vi "ExecuteSpeed.vi"(8 "Error In":errorcluster, 11 "RobotDriveDevRef":T1={"DevStatus"={"status"=FALSE, "code"=0, "source"=""}, "Motors[]"=[], "Square Inputs"=FALSE, "Max Output"=1.0}) -> (0 "Error Out":errorcluster)   [LabVIEW 2020]
uses:
  <vilib>/Rock Robotics/WPI/RobotDrive/WPI_RobotDriveDevRef.ctl
  <vilib>/Rock Robotics/WPI/MotorControl/WPI_MotorControlDeviceRef.ctl
  <vilib>/Rock Robotics/WPI/MotorControl/WPI_MotorControlType.ctl
  <vilib>/Rock Robotics/SystemInterfaces/DIO/FPGA_DIOPWMChannel.ctl
  <vilib>/Rock Robotics/WPI/PWM/WPI_PWMDeadband.ctl
  <vilib>/Rock Robotics/SystemInterfaces/DIO/FPGA_DIOChannel.ctl
  <vilib>/Rock Robotics/WPI/ThirdParty/JAS_Junk/TrajLib/PIDController_AtSetpoint.vi
  <vilib>/Rock Robotics/WPI/ThirdParty/JAS_Junk/TrajLib/PIDController_SetPIDF.vi
  <vilib>/Rock Robotics/WPI/ThirdParty/JAS_Junk/TrajLib/PIDController_SetDerivativeFilter.vi
  <vilib>/Rock Robotics/WPI/ThirdParty/JAS_Junk/TrajLib/PIDController_SetIntegratorRange.vi
  <vilib>/Rock Robotics/WPI/ThirdParty/JAS_Junk/TrajLib/PIDController_SetTolerancePandV.vi
  <vilib>/Rock Robotics/WPI/ThirdParty/JAS_Junk/TrajLib/PIDController_DisableContinousInput.vi
  <vilib>/Rock Robotics/WPI/ThirdParty/JAS_Junk/TrajLib/PIDController_EnableContinousInput.vi
  <vilib>/Rock Robotics/WPI/ThirdParty/JAS_Junk/TrajLib/PIDController_Reset.vi
  <vilib>/Rock Robotics/WPI/ThirdParty/JAS_Junk/TrajLib/PIDController_New.vi
  <vilib>/Rock Robotics/WPI/ThirdParty/JAS_Junk/TrajLib/PIDController_SetOutputLimits.vi
  <vilib>/Rock Robotics/WPI/ThirdParty/JAS_Junk/TrajLib/SlewRateLimiter_New.vi
  <vilib>/Rock Robotics/WPI/ThirdParty/JAS_Junk/TrajLib/SlewRateLimiter_Reset.vi
  <vilib>/Rock Robotics/WPI/ThirdParty/JAS_Junk/TrajLib/SlewRateLimiter_Calculate.vi
  <vilib>/Rock Robotics/WPI/ThirdParty/JAS_Junk/TrajLib/SlewRateLimiter_SetRate.vi
  <vilib>/Rock Robotics/WPI/ThirdParty/JAS_Junk/TrajLib/ControllerUtil_GetModulusError.vi
  <vilib>/Rock Robotics/WPI/ThirdParty/JAS_Junk/TrajLib/PIDController_NewPeriod.vi
  <vilib>/Rock Robotics/SystemInterfaces/NetworkCommunication/NetComm_UsageReport_report.vi
  DriveGlobals.vi
  <vilib>/Rock Robotics/WPI/ThirdParty/JAS_Junk/TrajLib/Util_GetTime.vi
  <vilib>/Rock Robotics/WPI/ThirdParty/JAS_Junk/TrajLib/Util_LibraryGlobals.vi
  <vilib>/Rock Robotics/WPI/ThirdParty/JAS_Junk/TrajLib/PIDController_AdvCalculate_FF_Sp_Pv.vi
  <vilib>/Rock Robotics/Network Tables/NT Write Numeric Array.vi
  <vilib>/Rock Robotics/WPI/ThirdParty/JAS_Junk/TrajLib/Trajectory_Library.lvlib
  <vilib>/Rock Robotics/WPI/DriverStation/WPI_DriverStationRobotMode2.ctl
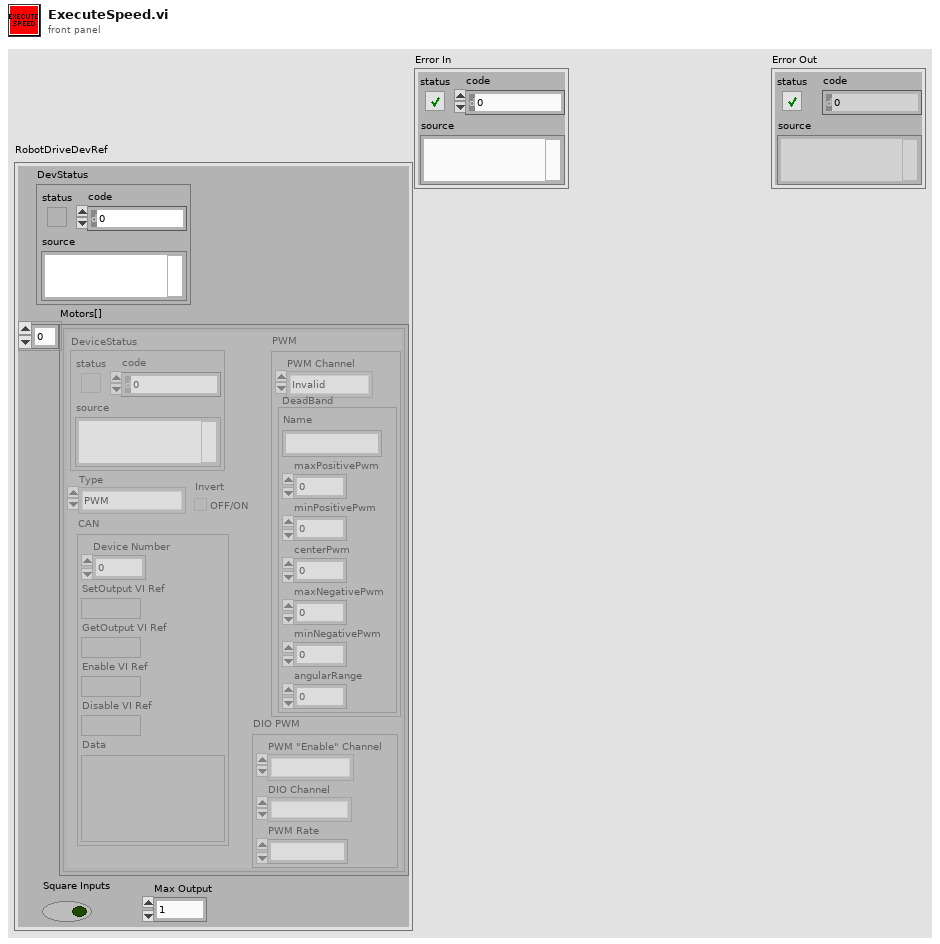
[diagram p1: front panel]
types:
  T1 = typedef "WPI_RobotDriveDevRef.ctl" = cluster{"DevStatus":errorcluster, "Motors[]":T2[], "Square Inputs":bool, "Max Output":dbl}
  T2 = typedef "WPI_MotorControlDeviceRef.ctl" = cluster{"DeviceStatus":errorcluster, "Type":T3, "PWM":cluster{"PWM Channel":T4, "DeadBand":T5}, "CAN":cluster{"Device Number":u8, "SetOutput VI Ref":variant, "GetOutput VI Ref":variant, "Enable VI Ref":variant, "Disable VI Ref":variant, "Data":variant}, "Invert":bool, "DIO PWM":cluster{"PWM \"Enable\" Channel":T4, "DIOChannel":T6, "PWM Rate":dbl}}
  T3 = typedef "WPI_MotorControlType.ctl" = enum16{"PWM", "CAN", "DIO PWM"}
  T4 = typedef "FPGA_DIOPWMChannel.ctl" = enum8{"PWM 0", "PWM 1", "PWM 2", "PWM 3", "PWM 4", "PWM 5", "PWM 6", "PWM 7", "PWM 8", "PWM 9", "PWM MXP 0", "PWM MXP 1", "PWM MXP 2", "PWM MXP 3", "PWM MXP 4", "PWM MXP 5", "PWM MXP 6", "PWM MXP 7", "PWM MXP 8", "PWM MXP 9", "Invalid"}
  T5 = typedef "WPI_PWMDeadband.ctl" = cluster{"Name":string, "maxPositivePwm":i32, "minPositivePwm":i32, "centerPwm":i32, "maxNegativePwm":i32, "minNegativePwm":i32, "angularRange":u16}
  T6 = typedef "FPGA_DIOChannel.ctl" = enum8{"DIO 0", "DIO 1", "DIO 2", "DIO 3", "DIO 4", "DIO 5", "DIO 6", "DIO 7", "DIO 8", "DIO 9", "DIO MXP 0", "DIO MXP 1", "DIO MXP 2", "DIO MXP 3", "DIO MXP 4", "DIO MXP 5", "DIO MXP 6", "DIO MXP 7", "DIO MXP 8", "DIO MXP 9", "DIO MXP 10", "DIO MXP 11", "DIO MXP 12", "DIO MXP 13", "DIO MXP 14", "DIO MXP 15", "SPI Port CS1", "SPI Port CS2", "SPI Port CS3", "SPI Port MISO", "SPI Port MOSI", "Invalid"}
  T7 = typedef "WPI_DriverStationRobotMode2.ctl" = enum16{"Autonomous Disabled", "Autonomous Enabled", "Teleop Disabled", "Teleop Enabled", "Disconnected", "Finish", "Test Disabled", "Test Enabled", "Emergency Stopped"}
  T8 = typedef "Trajectory_Library.lvlib/PID_ADV_LIMITS.ctl" = cluster{"MaxInput":dbl, "MinInput":dbl, "Continuous":bool, "MaxOutput":dbl, "MinOutput":dbl}
  T9 = typedef "Trajectory_Library.lvlib/PID_ADV_TUNING.ctl" = cluster{"Kf":dbl, "Kp":dbl, "Ki":dbl, "Kd":dbl, "MaximumIntegral":dbl, "MinimumIntegral":dbl, "Filter Derivative":bool}
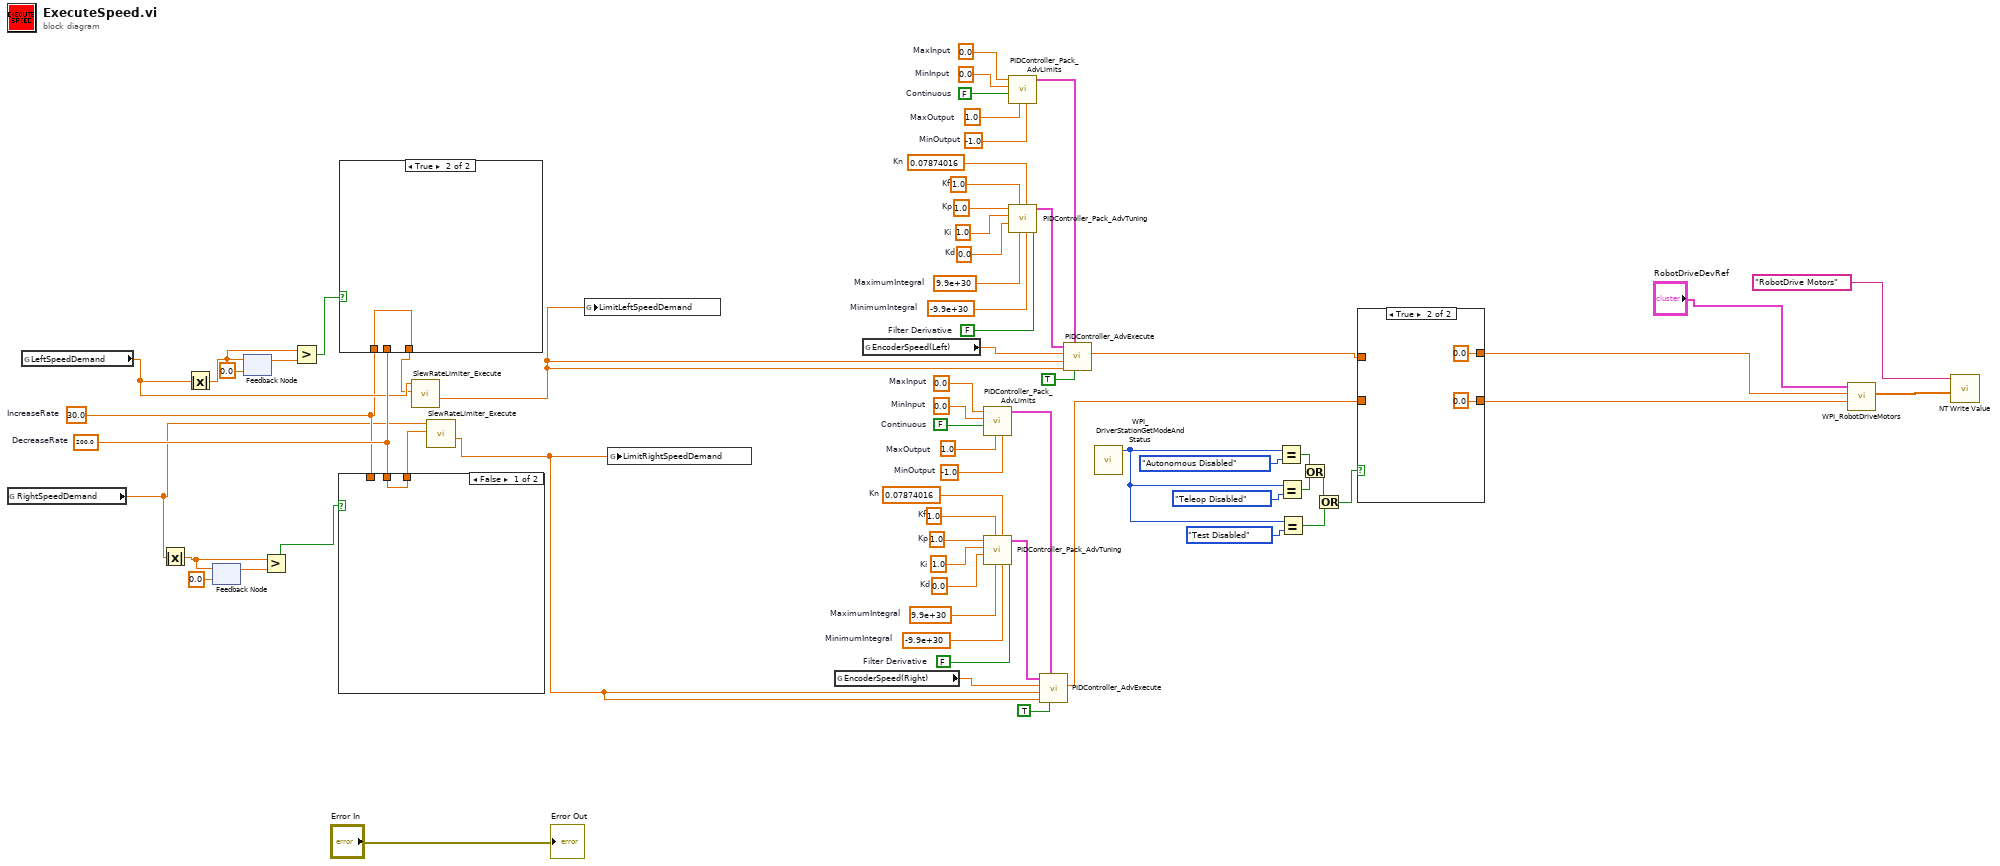
[diagram p0: block diagram]
diagram:
  w42 = 0.07874016  # Kn
  w41 = 1.0  # Kp
  w40 = 1.0  # Ki
  w39 = 0.0  # Kd
  w38 = 1.0  # Kf
  w37 = 9.9e+30  # MaximumIntegral
  w36 = -9.9e+30  # MinimumIntegral
  w35 = FALSE  # Filter Derivative
  w33 = 0.0  # MinInput
  w32 = FALSE  # Continuous
  w31 = 1.0  # MaxOutput
  w34 = -1.0  # MinOutput
  w30 = 0.0  # MaxInput
  w58 = 0.07874016  # Kn
  w57 = 1.0  # Kp
  w56 = 1.0  # Ki
  w55 = 0.0  # Kd
  w54 = 1.0  # Kf
  w53 = 9.9e+30  # MaximumIntegral
  w52 = -9.9e+30  # MinimumIntegral
  w51 = FALSE  # Filter Derivative
  w49 = 0.0  # MinInput
  w48 = FALSE  # Continuous
  w47 = 1.0  # MaxOutput
  w50 = -1.0  # MinOutput
  w46 = 0.0  # MaxInput
  w59 = 200.0  # DecreaseRate
  w18 = 30.0  # IncreaseRate
  n1 = global read "DriveGlobals.vi" "RightSpeedDemand"() -> (w16:dbl)
  n2 = global read "DriveGlobals.vi" "LeftSpeedDemand"() -> (w24:dbl)
  n3 = Absolute Value(x=w16) -> (abs(x)=w26:dbl)
  n4 = Absolute Value(x=w24) -> (abs(x)=w25:dbl)
  n5 = feedback #1(0.0 ("LeftSpeedDemand")) -> (w61:dbl)
  n6 = feedback-in #1(w26) -> ()
  n7 = feedback-in #2(w25) -> ()
  n8 = feedback #2(0.0 ("LeftSpeedDemand")) -> (w64:dbl)
  n9 = Greater?(x=w26, y=w61) -> (0:w23:bool)
  n10 = Greater?(x=w25, y=w64) -> (0:w63:bool)
  n11 = case shown="False" w23 {
    tunnel: w59 -> [w68 _]
    tunnel: w18 -> [_ w69]
    tunnel: [w68 w69] -> w17
    frame False {
    }
    frame True {
    }
  }
  n12 = case shown="True" w63 {
    tunnel: w18 -> [_ w71]
    tunnel: w59 -> [w70 _]
    tunnel: [w70 w71] -> w14
    frame False {
    }
    frame True {
    }
  }
  n13 = call <vilib>:"SlewRateLimiter_Execute.vi"("Rate"=w14, "Input"=w24) -> ("Output"=w15:dbl)  [unwired: 8 in, 1 out]
  n14 = call <vilib>:"SlewRateLimiter_Execute.vi"("Rate"=w17, "Input"=w16) -> ("Output"=w19:dbl)  [unwired: 8 in, 1 out]
  n15 = global write "DriveGlobals.vi" "LimitLeftSpeedDemand"(w15) -> ()
  n16 = global write "DriveGlobals.vi" "LimitRightSpeedDemand"(w19) -> ()
  n17 = global read "DriveGlobals.vi" "EncoderSpeed(Right)"() -> (w43:dbl)
  n18 = global read "DriveGlobals.vi" "EncoderSpeed(Left)"() -> (w27:dbl)
  n19 = call <vilib>:"PIDController_Pack_AdvLimits.vi"("MinOutput"=w50, "MaxOutput"=w47, "Continuous"=w48, "MinInput"=w49, "MaxInput"=w46) -> ("Adv PID Limits"=w44:T8)  [unwired: 6 in]
  n20 = call <vilib>:"PIDController_Pack_AdvTuning.vi"("Filter Derivative"=w51, "MinimumIntegral"=w52, "Kn"=w58, "MaximumIntegral"=w53, "Kf"=w54, "Kd"=w55, "Ki"=w56, "Kp"=w57) -> ("Adv PID Tuning"=w45:T9)  [unwired: 3 in]
  n21 = call <vilib>:"PIDController_Pack_AdvLimits.vi"("MinOutput"=w34, "MaxOutput"=w31, "Continuous"=w32, "MinInput"=w33, "MaxInput"=w30) -> ("Adv PID Limits"=w28:T8)  [unwired: 6 in]
  n22 = call <vilib>:"PIDController_Pack_AdvTuning.vi"("Filter Derivative"=w35, "MinimumIntegral"=w36, "Kn"=w42, "MaximumIntegral"=w37, "Kf"=w38, "Kd"=w39, "Ki"=w40, "Kp"=w41) -> ("Adv PID Tuning"=w29:T9)  [unwired: 3 in]
  n23 = call <vilib>:"PIDController_AdvExecute.vi"("Auto"=TRUE, "Adv PID Limits"=w44, "FF-FeedForward"=w19, "SP-SetPoint"=w19, "PV-Measurement"=w43, "Adv PID Tuning"=w45) -> ("CO-ControlOutput"=w4:dbl)  [unwired: 3 in, 2 out]
  n24 = call <vilib>:"PIDController_AdvExecute.vi"("Auto"=TRUE, "Adv PID Limits"=w28, "FF-FeedForward"=w15, "SP-SetPoint"=w15, "PV-Measurement"=w27, "Adv PID Tuning"=w29) -> ("CO-ControlOutput"=w5:dbl)  [unwired: 3 in, 2 out]
  n25 = call <vilib>:"WPI_DriverStationGetModeAndStatus.vi"() -> ("Robot Mode"=w10:T7)  [unwired: 10 in, 1 out]
  n26 = Equal?(x=w10, y=WPI_DriverStationRobotMode2."Autonomous Disabled" ("Robot Mode")) -> (x = y?=w8:bool)
  n27 = Equal?(x=w10, y=WPI_DriverStationRobotMode2."Teleop Disabled" ("Robot Mode")) -> (x = y?=w7:bool)
  n28 = Equal?(x=w10, y=WPI_DriverStationRobotMode2."Test Disabled" ("Robot Mode")) -> (x = y?=w6:bool)
  n29 = Or(x=w8, y=w7) -> (x .or. y?=w9:bool)
  n30 = Or(x=w9, y=w6) -> (x .or. y?=w1:bool)
  n31 = case shown="True" w1 {
    tunnel: w5 -> [w72 _]
    tunnel: w4 -> [w73 _]
    tunnel: [w73 0.0 ("CO-ControlOutput")] -> w3
    tunnel: [w72 0.0 ("CO-ControlOutput")] -> w2
    frame False {
    }
    frame True {
    }
  }
  n32 = call <vilib>:"WPI_RobotDriveMotors.vi"("RightSpeed"=w3, "LeftSpeed"=w2, "RobotDriveDevRef"="RobotDriveDevRef") -> ("Motor Values"=w67:dbl[])  [unwired: 6 in, 2 out]
  n33 = call-poly <vilib>:"NT Write Value.vi"("Numeric Array"=w67, "Name"="RobotDrive Motors") -> ()  [unwired: 9 in, 1 out]
  "Error Out" <- "Error In"
